vi "AlliGator Get Available Fitting Parameters.vi"(11 "Parameter Names":T1[](array[typedef])) -> (3 "Missing Parameter Names":T1[](array[typedef]))   [LabVIEW 2021, in "AlliGator Settings.lvlib"]
doc: "Returns list of parameters not in the <B>Parameter Names</B> list."
uses:
  AlliGator Settings.lvlib
  Fits/IRF(X)PSED/Decay Fit Parameters In List.ctl
  325204a7-54f9-4925-b933-958484244497.vi
  <userlib>/_OpenG.lib/array/array.llb/Filter 1D Array (I32)__ogtk.vi
  <userlib>/_OpenG.lib/array/array.llb/openg_array.lvlib
  Fits/Fits.lvlib
panel:
  in  "Fit Parameter used to access parameter name list":T1
  # "see the AlliGator License on the block diagram (Ctrl+E or Window:Show Block Diagram)"
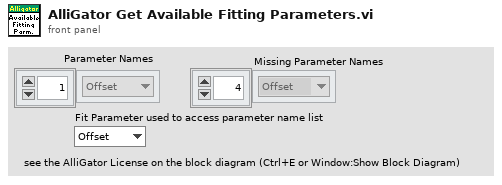
[diagram p1: front panel]
types:
  T1 = typedef "Fits.lvlib/Decay Fit Parameters In List.ctl" = enum16{"Offset", "Baseline", "A_1", "tau_1", "A_2", "tau_2"}
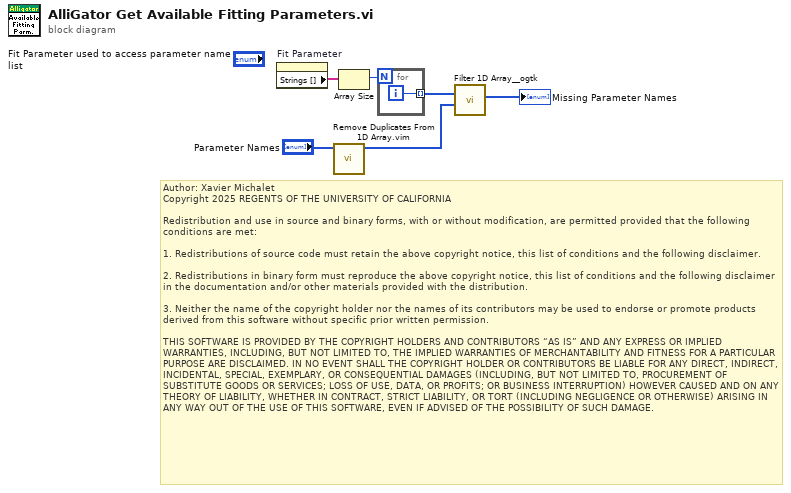
[diagram p0: block diagram]
diagram:
  # "Author: Xavier Michalet\nCopyright 2025 REGENTS OF THE UNIVERSITY OF CALIFORNIA\n\nRedistribution and use in source and binary forms, with or without modification, are permitted provided that the following conditions are met:\n\n1. Redistributions of source code must retain the above copyright notice, this list of conditions and the following disclaimer.\n\n2. Redistributions in binary form must reproduce the above copyright notice, this list of conditions and the following disclaimer in the documentation and/or other materials provided with the distribution.\n\n3. Neither the name of the copyright holder nor the names of its contributors may be used to endorse or promote products derived from this software without specific prior written permission.\n\nTHIS SOFTWARE IS PROVIDED BY THE COPYRIGHT HOLDERS AND CONTRIBUTORS “AS IS” AND ANY EXPRESS OR IMPLIED WARRANTIES, INCLUDING, BUT NOT LIMITED TO, THE IMPLIED WARRANTIES OF MERCHANTABILITY AND FITNESS FOR A PARTICULAR PURPOSE ARE DISCLAIMED. IN NO EVENT SHALL THE COPYRIGHT HOLDER OR CONTRIBUTORS BE LIABLE FOR ANY DIRECT, INDIRECT, INCIDENTAL, SPECIAL, EXEMPLARY, OR CONSEQUENTIAL DAMAGES (INCLUDING, BUT NOT LIMITED TO, PROCUREMENT OF SUBSTITUTE GOODS OR SERVICES; LOSS OF USE, DATA, OR PROFITS; OR BUSINESS INTERRUPTION) HOWEVER CAUSED AND ON ANY THEORY OF LIABILITY, WHETHER IN CONTRACT, STRICT LIABILITY, OR TORT (INCLUDING NEGLIGENCE OR OTHERWISE) ARISING IN ANY WAY OUT OF THE USE OF THIS SOFTWARE, EVEN IF ADVISED OF THE POSSIBILITY OF SUCH DAMAGE."
  n1 = property on="Fit Parameter" class="Enum (strict)"() -> ("Strings []"=w5:string[])  [unwired: 2 in, 2 out]
  n2 = call "Remove Duplicates From 1D Array.vim"("array"="Parameter Names") -> ("array with duplicates removed"=w2:T1[])  [unwired: 10 in]
  n3 = Array Size(array=w5) -> (size(s)=w4:i32)
  n4 = for {
    N: w4 -> [_]
    tunnel: [w7] -> w3 mode=indexing
    i -> [w7]
  }
  n5 = call-poly <userlib>:"Filter 1D Array__ogtk.vi"("items to filter"=w2, "array"=w3) -> ("filtered array"=→"Missing Parameter Names":i32[])  [unwired: 4 in, 1 out]
